vi "Main.vi"(11 "Module Admin":refnum<class "Delacor_lib_QMH_Module Admin.lvclass">) -> ()   [LabVIEW 2024, in "EtherCAT Model.lvlib"]
doc: "This template is based off of the Queued Message Handler design pattern and the Queued Message Handler project template that ships with LabVIEW.\n\nThe main difference is that the queue is private to this module and communication between modules is performed via Broadcast and Request events.\n\nRequest events are wrapped in public API methods and are handled in the Event Handling Loop (EHL) of this VI. Any module can register for Broadcast events sent by this module. The EHL generates messages based on user interface actions.\n\nThe Message Handling Loop (MHL) processes messages generated by the EHL, or by other messages. The messages are string values, so new messages can be added easily to the Message Cases case structure in the MHL. Each message cluster can also provide an optional value for Message Data, which is a variant that can be converted to whatever message-specific data is required.\n_____\nBased on DQMH Project Template 7.0.1.1316."
uses:
  EtherCAT Model.lvlib
  <vilib>/Delacor/Delacor QMH/Libraries/Module Admin_class/Delacor_lib_QMH_Module Admin.lvclass
  EtherCAT Configuration.ctl
  Module Data--cluster.ctl
  Write Context Typedef.ctl
  EtherCAT Output Data Frame.ctl
  <vilib>/Delacor/Delacor QMH/Libraries/Message Queue_class/Delacor_lib_QMH_Message Queue.lvclass/Delacor_lib_QMH_Message Queue.ctl
  Stop Argument--cluster.ctl
  <vilib>/Delacor/Delacor QMH/Libraries/Module Admin_class/Delacor_lib_QMH_Module Admin.lvclass/Delacor_lib_QMH_Module Admin.ctl
  Load Configuration Argument--cluster.ctl
  Load Configuration (Reply Payload)--cluster.ctl
  Start Connection Argument--cluster.ctl
  Start Connection (Reply Payload)--cluster.ctl
  Close Connection Argument--cluster.ctl
  Close Connection (Reply Payload)--cluster.ctl
  Write U16 Argument--cluster.ctl
  Write U16 (Reply Payload)--cluster.ctl
  Write I16 Argument--cluster.ctl
  Write I16 (Reply Payload)--cluster.ctl
  <vilib>/Utility/miscctls.llb/LVPointTypeDef.ctl
  <instrlib>/_Ackermann Automation/EtherCAT Lib/EcatLib/TypeDefs/EnumBusState.ctl
  <instrlib>/_Ackermann Automation/EtherCAT Lib/EcatLib/TypeDefs/ClusterNetworkAdapters.ctl
  <instrlib>/_Ackermann Automation/EtherCAT Lib/EcatLib/TypeDefs/ClusterTargetConnectionWin.ctl
  <vilib>/Delacor/Delacor QMH/Libraries/Message Queue_class/Delacor_lib_QMH_Enqueue Message (Single).vi
  <vilib>/Delacor/Delacor QMH/Libraries/Module Admin_class/Delacor_lib_QMH_Get External Launch.vi
  <instrlib>/_Ackermann Automation/EtherCAT Lib/EcatLib/Conversion/ConvertU16ToFrameSingle.vi
  <instrlib>/_Ackermann Automation/EtherCAT Lib/EcatLib/Conversion/ConvertI16ToFrameSingle.vi
  <vilib>/Delacor/Delacor QMH/Libraries/Message Queue_class/Delacor_lib_QMH_Message Queue.lvclass
  <instrlib>/_Ackermann Automation/EtherCAT Lib/EcatLib/EthercatLib.lvlib
panel:
  out "Setup":T1
  out "EtherCAT Ref":u64
  out "error out":errorcluster
  out "Status":string
  in  "Simulate MHL Error":bool
  in  "Simulate EHL Error":bool
  # "Other processes communicate with this Module via its Public API (wrappers for its Request Events).\n\nThis Module communicates with other processes via its Broadcast Events.\nAny process that wants to receive these messages can register for this module's Broadcast events."
  # "Local Variable"
  # "This template is for the DQMH framework. See the block diagram for more information on how to use this template."
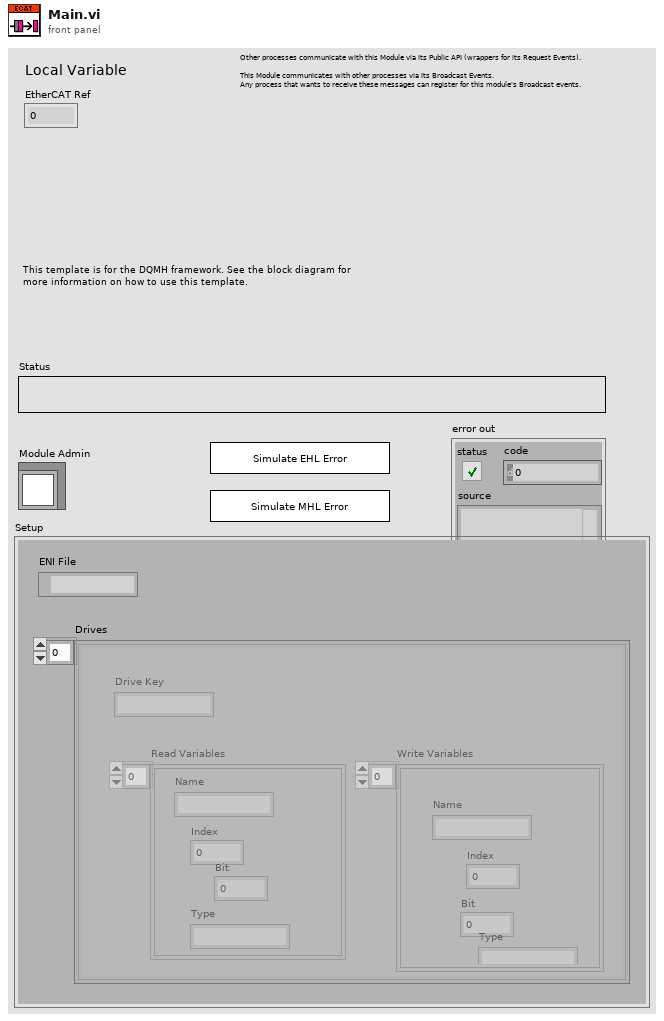
[diagram p1: front panel]
types:
  T1 = typedef "EtherCAT Configuration.ctl" = cluster{"ENI File":path, "Drives":cluster{"Drive Key":string, "Read Variables":cluster{"Name":string, "Index":i32, "Bit":u8, "Type":string}[], "Write Variables":cluster{"Name":string, "Index":i32, "Bit":u8, "Type":string}[]}[]}
  T2 = typedef "EtherCAT Model.lvlib/Request Events--cluster.ctl" = cluster{"Stop Module":refnum<user-event>, "Show Panel":refnum<user-event>, "Hide Panel":refnum<user-event>, "Get Module Execution Status":refnum<user-event>, "Show Diagram":refnum<user-event>, "Load Configuration":refnum<user-event>, "Start Connection":refnum<user-event>, "Close Connection":refnum<user-event>, "Private":cluster{"Start Read Timer Loop":refnum<user-event>, "Stop Read Timer Loop":refnum<user-event>, "Read Single Frame":refnum<user-event>}, "Write U16":refnum<user-event>, "Write I16":refnum<user-event>}
  T3 = typedef "EtherCAT Model.lvlib/Module Data--cluster.ctl" = cluster{"Status":string, "Setup":T1, "EtherCAT Connection":bool, "Write Map":T4, "EtherCAT Output Frame":T5}
  T4 = typedef "EtherCAT Model.lvlib/Write Context Typedef.ctl" = map{string, cluster{"Index":i32, "Bit":u8, "Type":string}}
  T5 = typedef "EtherCAT Model.lvlib/EtherCAT Output Data Frame.ctl" = u8[]
  T6 = enum32{"invalid lock state", "Not Locked", "Locked (No Password)", "Password-protected"}
  T7 = typedef "EtherCAT Model.lvlib/Stop Argument--cluster.ctl" = cluster{"Origin":string, "Exit via Stop Module Req?":bool, "Wait for Module to stop?":bool}
  T8 = typedef "EtherCAT Model.lvlib/Load Configuration Argument--cluster.ctl" = cluster{"Setup":T1, "Wait Notifier":refnum<notifier>, "wait for reply":bool}
  T9 = typedef "EtherCAT Model.lvlib/Start Connection Argument--cluster.ctl" = cluster{"Wait Notifier":refnum<notifier>, "wait for reply":bool}
  T10 = typedef "EtherCAT Model.lvlib/Close Connection Argument--cluster.ctl" = cluster{"Wait Notifier":refnum<notifier>, "wait for reply":bool}
  T11 = typedef "EtherCAT Model.lvlib/Write U16 Argument--cluster.ctl" = cluster{"Drive":string, "Variable":string, "Data":u16, "Wait Notifier":refnum<notifier>, "wait for reply":bool}
  T12 = typedef "EtherCAT Model.lvlib/Write I16 Argument--cluster.ctl" = cluster{"Drive":string, "Variable":string, "Data":i16, "Wait Notifier":refnum<notifier>, "wait for reply":bool}
  T13 = typedef "LVPointTypeDef.ctl" = cluster{"Horizontal":i16, "Vertical":i16}
  T14 = enum32{"Invalid", "Standard", "Closed", "Hidden", "Minimized", "Maximized"}
  T15 = typedef "EtherCAT Model.lvlib/Load Configuration (Reply Payload)--cluster.ctl" = cluster{"error":errorcluster}
  T16 = typedef "EtherCAT Model.lvlib/Start Connection (Reply Payload)--cluster.ctl" = cluster{"error":errorcluster}
  T17 = typedef "EthercatLib.lvlib/ClusterTargetConnectionWin.ctl" = cluster{"Target IP":string, "RPC Port":u32}
  T18 = typedef "EthercatLib.lvlib/ClusterNetworkAdapters.ctl" = cluster{"Primary":string, "Cable Redundancy":string}
  T19 = typedef "EtherCAT Model.lvlib/Close Connection (Reply Payload)--cluster.ctl" = cluster{"error":errorcluster}
  T20 = typedef "EtherCAT Model.lvlib/Write U16 (Reply Payload)--cluster.ctl" = cluster{"error":errorcluster}
  T21 = typedef "EtherCAT Model.lvlib/Write I16 (Reply Payload)--cluster.ctl" = cluster{"error":errorcluster}
  T22 = typedef "EthercatLib.lvlib/EnumBusState.ctl" = enum16{"Init", "PreOp", "Boot", "SafeOp", "Op"}
  T23 = typedef "EthercatLib.lvlib/ClusterBusSetup.ctl" = cluster{"Count Slaves Online":u32, "Count Slaves Configured":u32, "Process Data Bytes Input":u32, "Process Data  Bytes Output":u32, "Distributed Clocks":bool, "Hot Connect":bool}
  T24 = cluster{"Drive Key":string, "Read Variables":cluster{"Name":string, "Index":i32, "Bit":u8, "Type":string}[], "Write Variables":cluster{"Name":string, "Index":i32, "Bit":u8, "Type":string}[]}[]
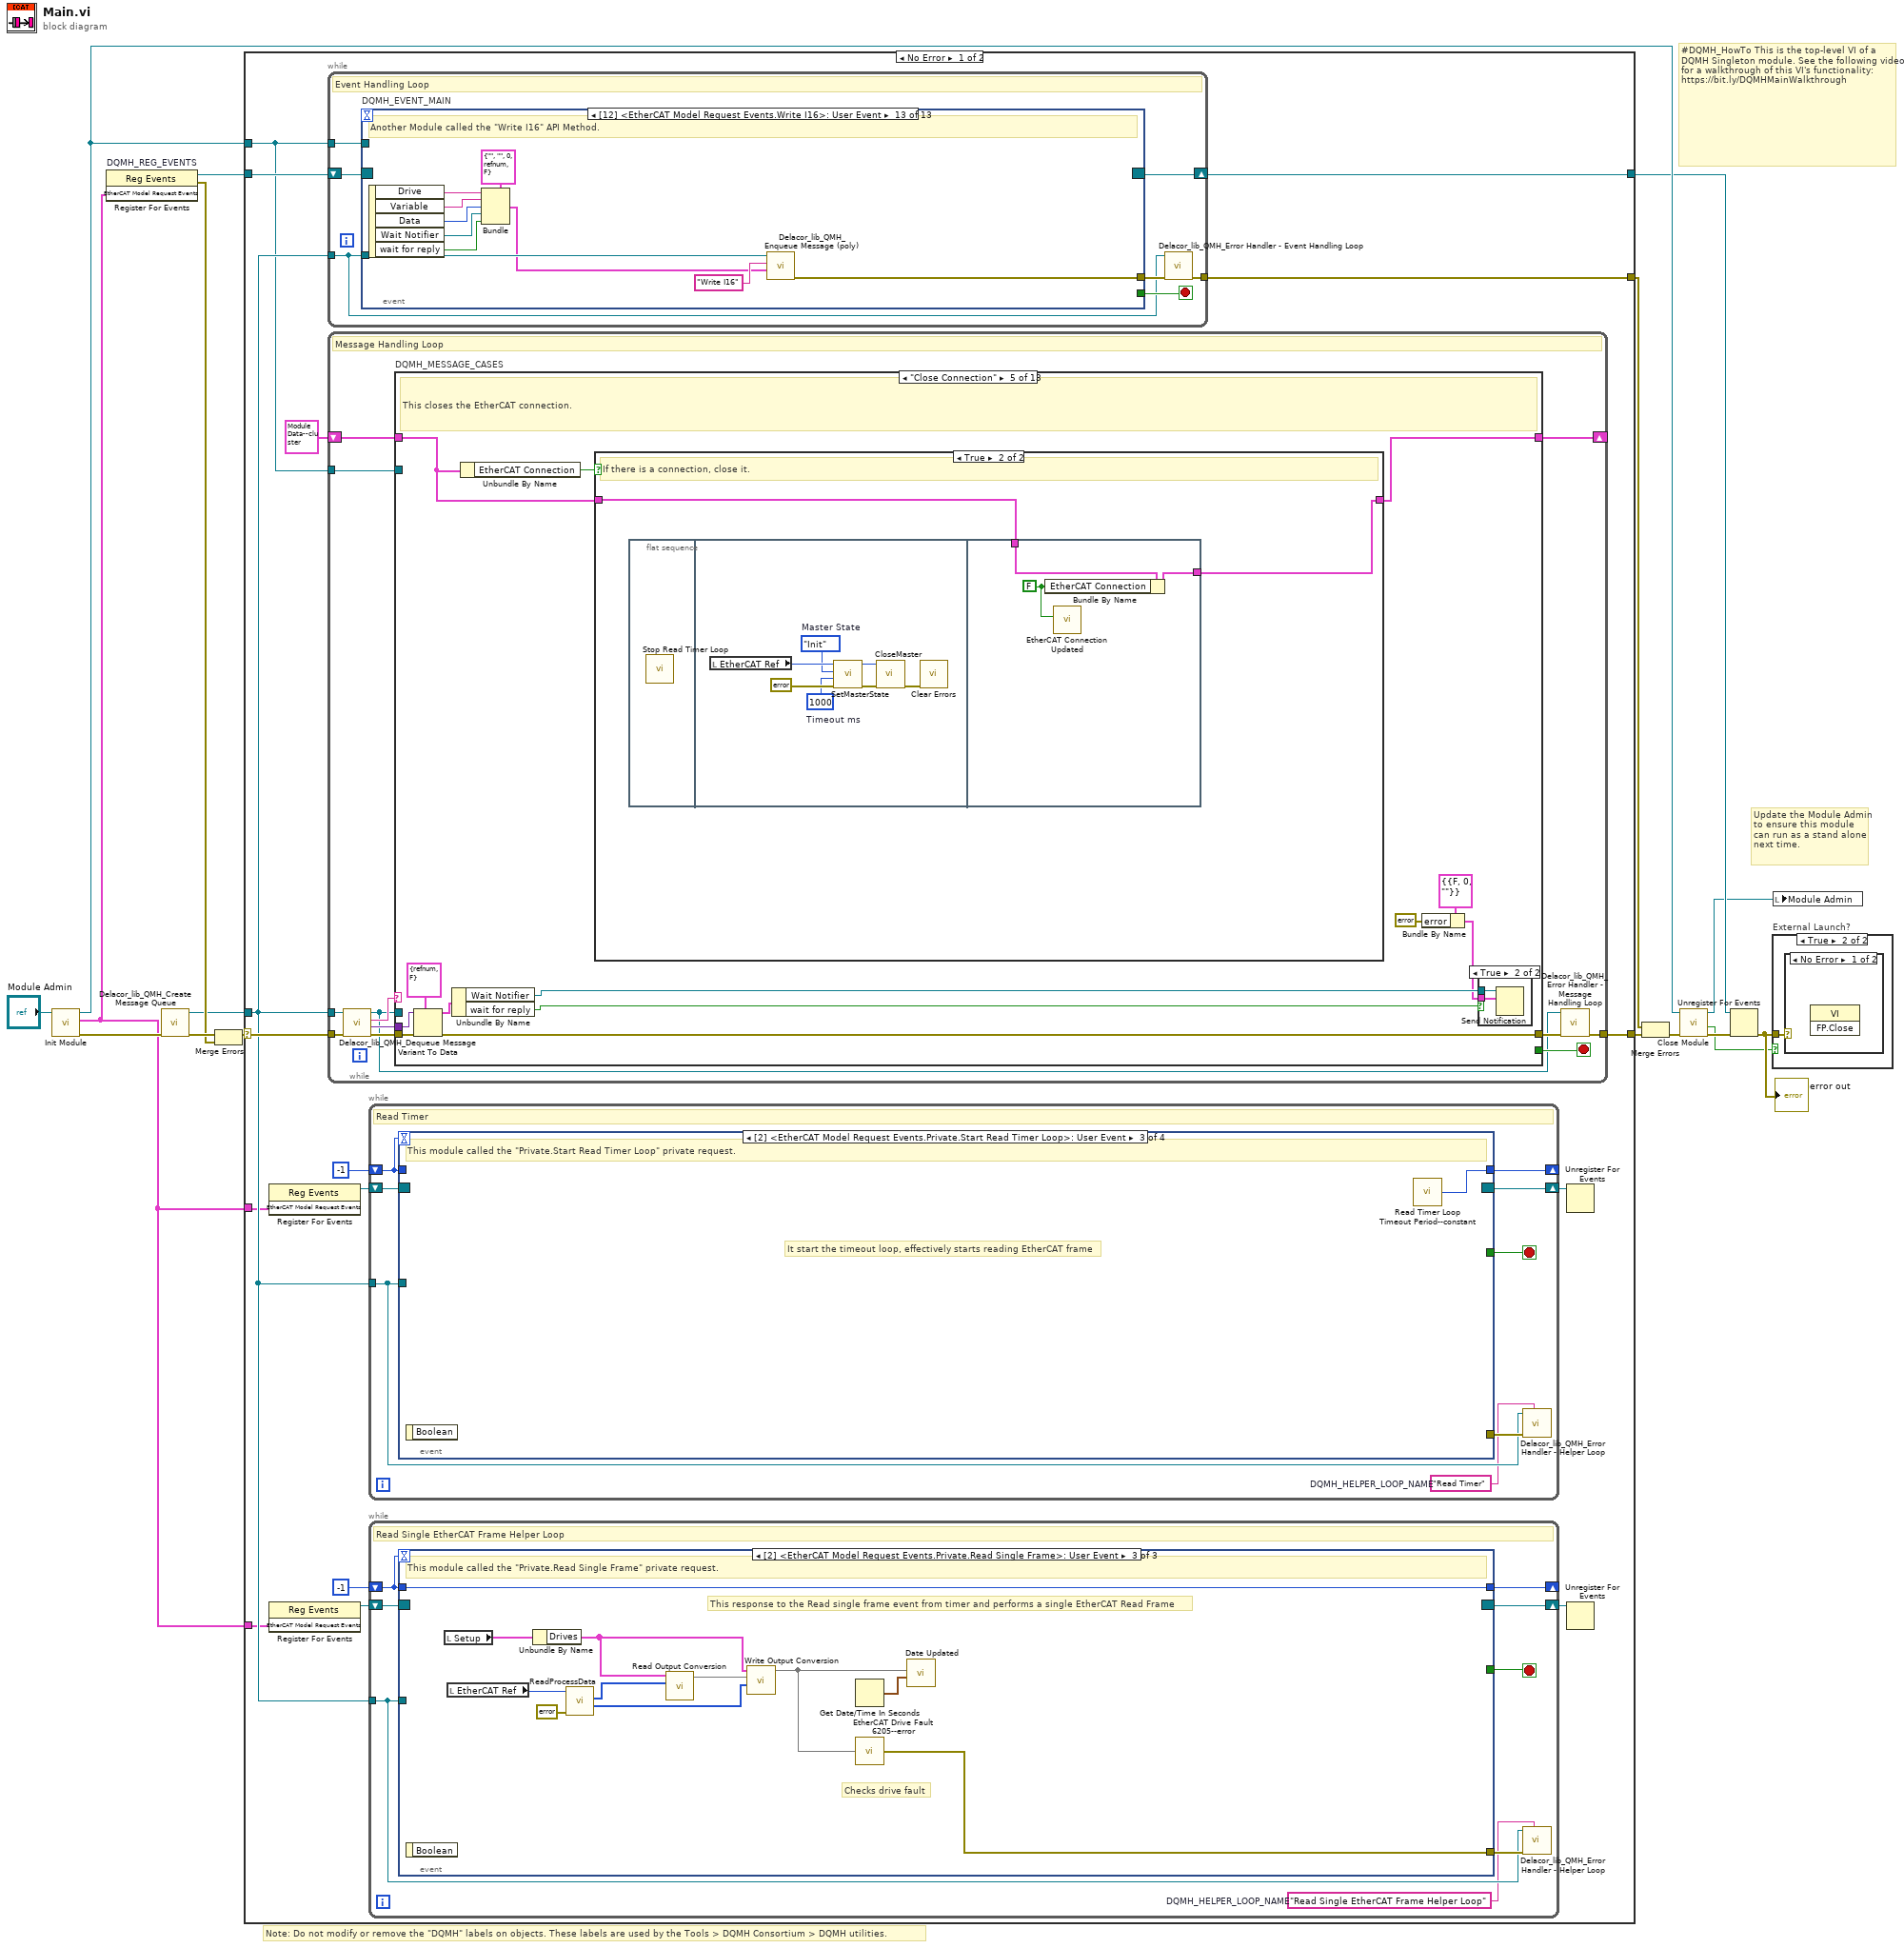
[diagram p0: block diagram]
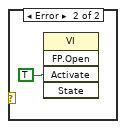
[diagram p3: hidden frame]
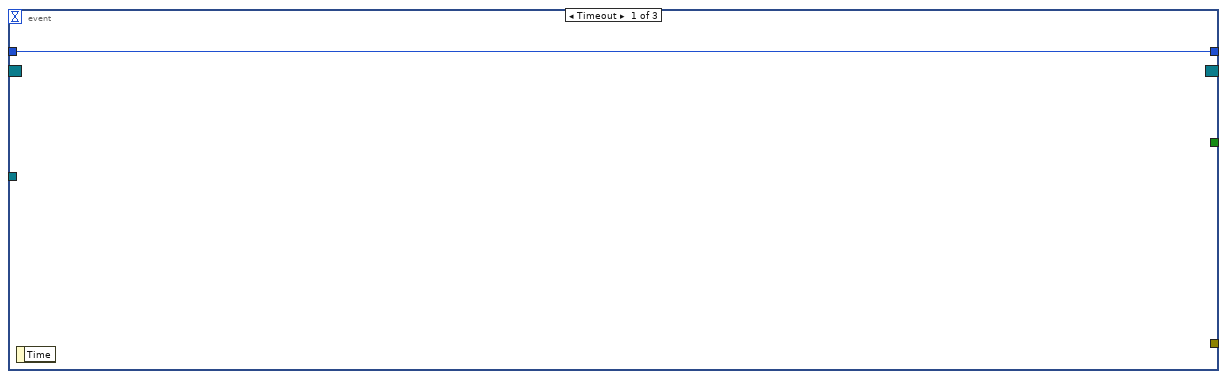
[diagram p4: hidden frame]
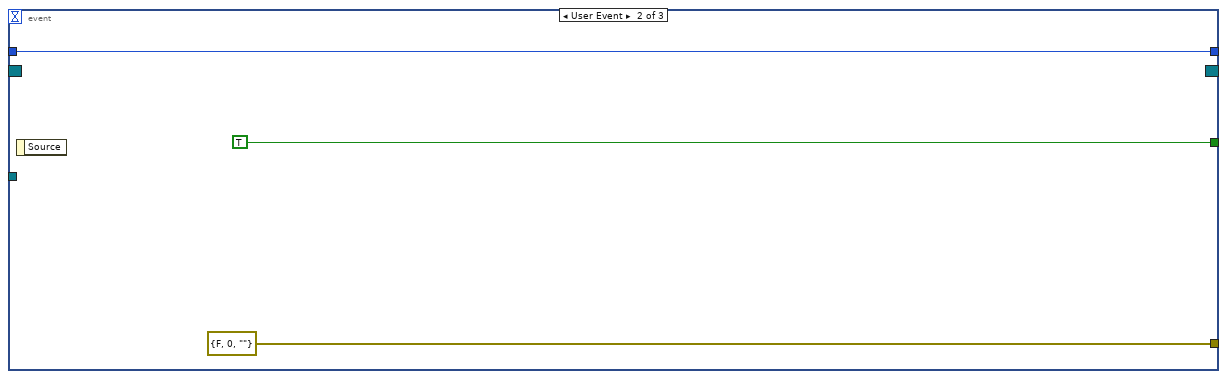
[diagram p5: hidden frame]
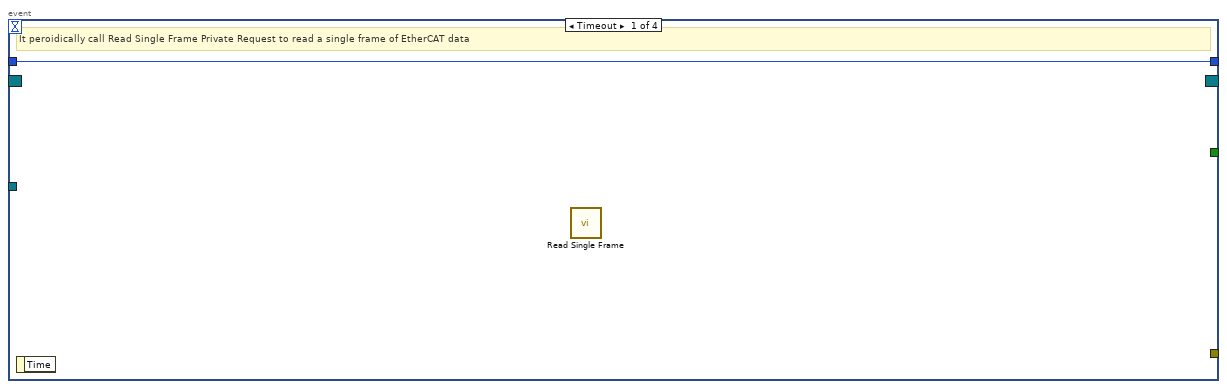
[diagram p6: hidden frame]
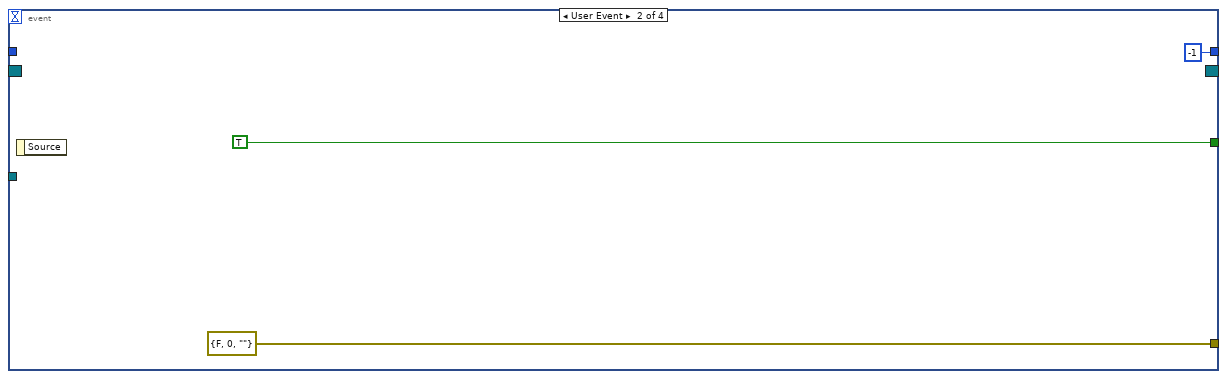
[diagram p7: hidden frame]
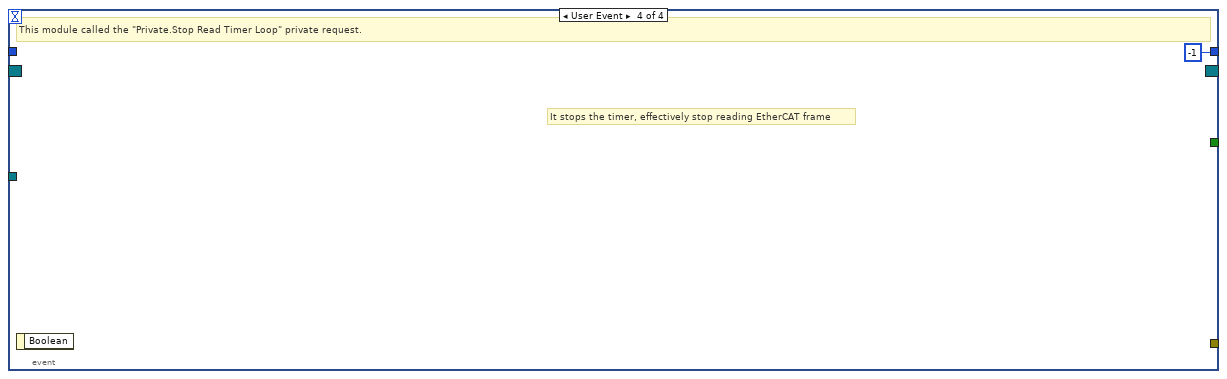
[diagram p8: hidden frame]
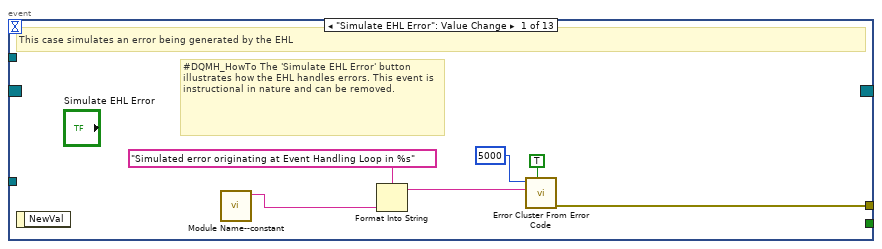
[diagram p9: hidden frame]
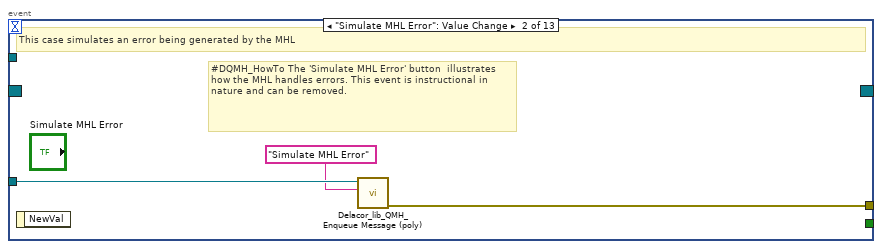
[diagram p10: hidden frame]
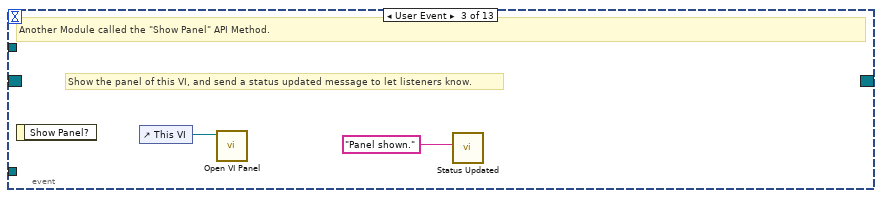
[diagram p11: hidden frame]
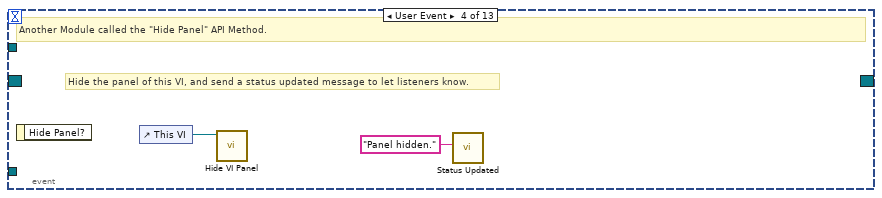
[diagram p12: hidden frame]
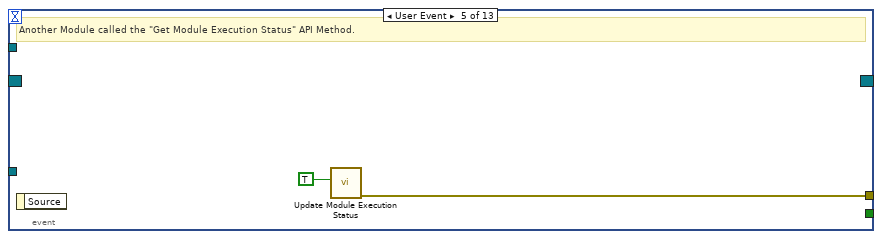
[diagram p13: hidden frame]
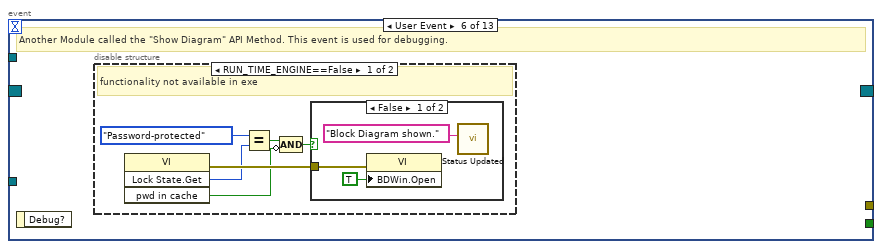
[diagram p14: hidden frame]
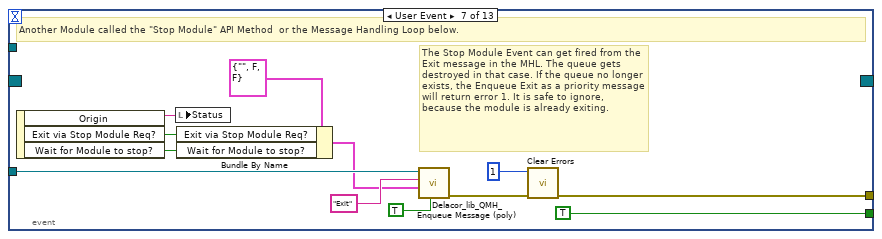
[diagram p17: hidden frame]
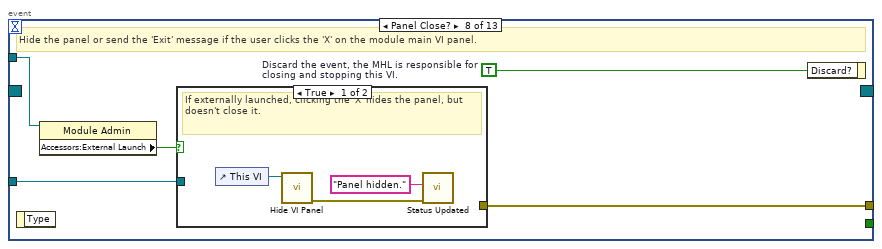
[diagram p18: hidden frame]
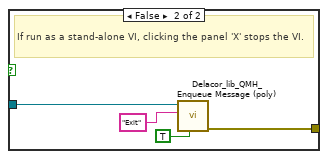
[diagram p19: hidden frame]
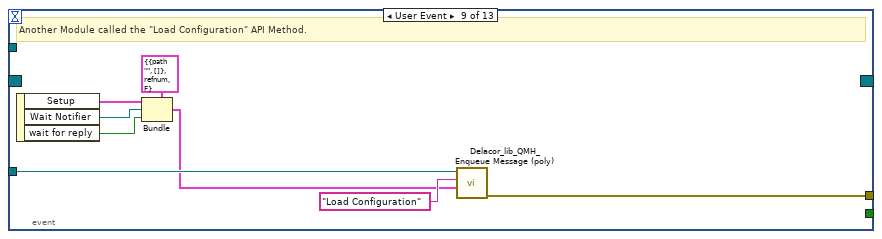
[diagram p20: hidden frame]
diagram:
  # "#DQMH_HowTo This is the top-level VI of a DQMH Singleton module. See the following video for a walkthrough of this VI's functionality: https://bit.ly/DQMHMainWalkthrough"
  # "Note: Do not modify or remove the \"DQMH\" labels on objects. These labels are used by the Tools > DQMH Consortium > DQMH utilities."
  # "Update the Module Admin to ensure this module can run as a stand alone next time."
  n1 = call "Init Module.vi"("Singleton Module Admin in"="Module Admin") -> ("error out"=w16:errorcluster, "EtherCAT Model Request Events"=w1:T2, "Singleton Module Admin out"=w8:refnum<class "Delacor_lib_QMH_Module Admin.lvclass">)  [unwired: 8 in]
  n2 = register-events "DQMH_REG_EVENTS"(w1) -> (reference out=w6:refnum<event-registration>, error out=w9:errorcluster)  [unwired: 2 in]
  n3 = call <vilib>:"Delacor_lib_QMH_Create Message Queue.vi"("error in"=w16) -> ("error out"=w11:errorcluster, "Message Queue"=w5:refnum<class "Delacor_lib_QMH_Message Queue.lvclass">)  [unwired: 9 in]
  n4 = Merge Errors(w11, w9) -> (w10:errorcluster)
  n5 = case shown="No Error" w10 {
    selector: w10 -> [w31 w489]
    tunnel: [w33 w488] -> w17
    tunnel: [w30 w487] -> w7
    tunnel: w6 -> [w28 w487]
    tunnel: w5 -> [w27 w482]
    tunnel: [w32 _] -> w14
    tunnel: w8 -> [w26 w483]
    tunnel: w1 -> [w25 _]
    tunnel: w1 -> [w21 _]
    frame No Error {
      n6 = register-events ("DQMH_HELPER_REGFOREVENTS")(w25) -> (reference out=w23:refnum<event-registration>)  [unwired: 2 in, 1 out]
      n7 = register-events ("DQMH_HELPER_REGFOREVENTS")(w21) -> (reference out=w19:refnum<event-registration>)  [unwired: 2 in, 1 out]
      n8 = while {
        tunnel: w27 -> [w71]
        shift-right: [w74] -> w30
        shift-left: w28 -> [w75]
        tunnel: [w76] -> w32
        tunnel: w26 -> [w72]
        stop <- w73 stop-if-true
        # "Event Handling Loop"
        n9 = event "DQMH_EVENT_MAIN" shown="[12] <EtherCAT Model Request Events.Write I16>: User Event" {
          selector: w75 -> [_ _ _ _ _ _ _ _ _ _ _ _ _]
          dyn-events: [_ _ _ _ _ _ _ _ _ _ _ _ _] -> w74
          timeout: _ -> [_ _ _ _ _ _ _ _ _ _ _ _ _]
          tunnel: [_ _ _ _ _ _ TRUE ("Discard?") _ _ _ _ _ _] -> w73
          tunnel: w71 -> [_ w85 _ _ _ _ w109 w116 w133 w140 w147 w157 w167]
          tunnel: [w83 w86 _ _ w92 _ w112 w118 w126 w134 w141 w148 w158] -> w77
          tunnel: w72 -> [_ _ _ _ _ _ _ w115 _ _ _ _ _]
          event "Simulate EHL Error": Value Change {
            # "#DQMH_HowTo The 'Simulate EHL Error' button  illustrates how the EHL handles errors. This event is instructional in nature and can be removed."
            # "This case simulates an error being generated by the EHL"
            n10 = event-data() -> ()  [unwired: 1 in, 1 out]
            n11 = call "Module Name--constant.vi"() -> ("Module Name"=w80:string)  [unwired: 11 in]
            n12 = Format Into String(format string="Simulated error originating at Event Handling Loop in %s", w80) -> (resulting string=w81:string)  [unwired: 2 in, 1 out]
            n13 = call <vilib>:"Error Cluster From Error Code.vi"("show call chain? (False)"=TRUE, "error message (\"\")"=w81, "error code (0)"=5000) -> ("error out"=w83:errorcluster)  [unwired: 6 in]
          }
          event "Simulate MHL Error": Value Change {
            # "#DQMH_HowTo The 'Simulate MHL Error' button  illustrates how the MHL handles errors. This event is instructional in nature and can be removed."
            # "This case simulates an error being generated by the MHL"
            n14 = event-data() -> ()  [unwired: 1 in, 1 out]
            n15 = call-poly <vilib>:"Delacor_lib_QMH_Enqueue Message (poly).vi"("Message"="Simulate MHL Error", "Message Queue in"=w85) -> ("error out"=w86:errorcluster)  [unwired: 8 in, 1 out]
          }
          event User Event {
            # "Show the panel of this VI, and send a status updated message to let listeners know."
            # "Another Module called the \"Show Panel\" API Method."
            n16 = event-data() -> ()  [unwired: 1 in, 1 out]
            n17 = control-ref of="This VI"() -> (w88:refnum<vi>)
            n18 = call "Open VI Panel.vi"("VI"=w88) -> ()  [unwired: 10 in, 1 out]
            n19 = call "Status Updated.vi"("Status"="Panel shown." ("format string")) -> ()  [unwired: 10 in, 1 out]
          }
          event User Event {
            # "Hide the panel of this VI, and send a status updated message to let listeners know."
            # "Another Module called the \"Hide Panel\" API Method."
            n20 = event-data() -> ()  [unwired: 1 in, 1 out]
            n21 = control-ref of="This VI"() -> (w90:refnum<vi>)
            n22 = call "Hide VI Panel.vi"("VI"=w90) -> ()  [unwired: 10 in, 1 out]
            n23 = call "Status Updated.vi"("Status"="Panel hidden." ("format string")) -> ()  [unwired: 10 in, 1 out]
          }
          event User Event {
            # "Another Module called the \"Get Module Execution Status\" API Method."
            n24 = event-data() -> ()  [unwired: 1 in, 1 out]
            n25 = call "Update Module Execution Status.vi"("Running?"=TRUE) -> ("error out"=w92:errorcluster)  [unwired: 10 in]
          }
          event User Event {
            # "Another Module called the \"Show Diagram\" API Method. This event is used for debugging."
            n26 = event-data() -> ()  [unwired: 1 in, 1 out]
            n27 = disable-structure shown="RUN_TIME_ENGINE==False" {
              frame condition #0 (active) {
                # "functionality not available in exe"
                n28 = invoke on="Invoke Node" class="VI" method="Lock State.Get"() -> (error out=w98:errorcluster, "Get Lock State"=w97:T6, "pwd in cache"=w94:bool)  [unwired: 4 in, 1 out]
                n29 = Equal?(x=T6."Password-protected", y=w97) -> (x = y?=w95:bool)
                n30 = Compound Arithmetic op=AND(w95, invert w94) -> (w93:bool)
                n31 = case shown="False" w93 {
                  tunnel: w98 -> [w101 _]
                  frame False {
                    n32 = property on="Property Node" class="VI"(error in=w101, "BDWin.Open"=TRUE ("Block Diagram Window:Open")) -> ()  [unwired: 1 in, 2 out]
                    n33 = call "Status Updated.vi"("Status"="Block Diagram shown." ("format string")) -> ()  [unwired: 10 in, 1 out]
                  }
                  frame True {
                    # "Password-protected VI, and the password is not in the cache. Do not show the diagram."
                  }
                }
              }
              frame condition #1 {
              }
            }
          }
          event User Event {
            # "The Stop Module Event can get fired from the Exit message in the MHL. The queue gets destroyed in that case. If the queue no longer exists, the Enqueue Exit as a priority message will return error 1. It is safe to ignore, because the module is already exiting."
            # "Another Module called the \"Stop Module\" API Method  or the Message Handling Loop below."
            n34 = event-data() -> ("Origin"=w108:string, "Exit via Stop Module Req?"=w104:bool, "Wait for Module to stop?"=w103:bool)  [unwired: 1 in]
            n35 = local write "Status"(w108) -> ()
            n36 = Bundle By Name(cluster=T7 {"Origin"="", "Exit via Stop Module Req?"=FALSE, "Wait for Module to stop?"=FALSE} ("Stop Argument"), "Exit via Stop Module Req?"=w104, "Wait for Module to stop?"=w103) -> (w102:T7)
            n37 = call-poly <vilib>:"Delacor_lib_QMH_Enqueue Message (poly).vi"("Priority Message? (F)"=TRUE, "Message Data"=w102, "Message"="Exit", "Message Queue in"=w109) -> ("error out"=w113:errorcluster)  [unwired: 6 in, 1 out]
            n38 = call <vilib>:"Clear Errors.vi"("error in (no error)"=w113, "specific error code to clear (0: all)"=1) -> ("error out"=w112:errorcluster)  [unwired: 4 in, 1 out]
          }
          event Panel Close? {
            w117 = TRUE  # Discard the event, the MHL is responsible for closing and stopping this VI.
            # "Hide the panel or send the 'Exit' message if the user clicks the 'X' on the module main VI panel."
            n39 = event-data() -> ()  [unwired: 1 in, 1 out]
            n40 = property on="Property Node" class="Module Admin"(reference=w115) -> ("Accessors:External Launch"=w114:bool)  [unwired: 1 in, 2 out]
            n41 = case shown="True" w114 {
              tunnel: w116 -> [_ w124]
              tunnel: [_ w125] -> w118
              frame True {
                # "If externally launched, clicking the 'X' hides the panel, but doesn't close it."
                n42 = control-ref of="This VI"() -> (w121:refnum<vi>)
                n43 = call "Hide VI Panel.vi"("VI"=w121) -> ("error out"=w119:errorcluster)  [unwired: 10 in]
                n44 = call "Status Updated.vi"("error in"=w119, "Status"="Panel hidden." ("format string")) -> ()  [unwired: 9 in, 1 out]
              }
              frame False {
                # "If run as a stand-alone VI, clicking the panel 'X' stops the VI."
                n45 = call-poly <vilib>:"Delacor_lib_QMH_Enqueue Message (poly).vi"("Priority Message? (F)"=TRUE, "Message"="Exit", "Message Queue in"=w124) -> ("error out"=w125:errorcluster)  [unwired: 7 in, 1 out]
              }
            }
            n46 = event-data ("Event Filter Node")("Discard?"=w117) -> ()  [unwired: 1 in, 1 out]
          }
          event User Event {
            # "Another Module called the \"Load Configuration\" API Method."
            n47 = event-data() -> ("Setup"=w129:T1, "Wait Notifier"=w128:refnum<notifier>, "wait for reply"=w127:bool)  [unwired: 1 in]
            n48 = Bundle(cluster=T8 {"Setup"={"ENI File"=path "", "Drives"=[]}, "Wait Notifier"=refnum, "wait for reply"=FALSE} ("Load Configuration Argument"), "Setup"=w129, "Wait Notifier"=w128, "wait for reply"=w127) -> (w130:T8)
            n49 = call-poly <vilib>:"Delacor_lib_QMH_Enqueue Message (poly).vi"("Message Data"=w130, "Message"="Load Configuration", "Message Queue in"=w133) -> ("error out"=w126:errorcluster)  [unwired: 7 in, 1 out]
          }
          event User Event {
            # "Another Module called the \"Start Connection\" API Method."
            n50 = event-data() -> ("Wait Notifier"=w136:refnum<notifier>, "wait for reply"=w135:bool)  [unwired: 1 in]
            n51 = Bundle(cluster=T9 {"Wait Notifier"=refnum, "wait for reply"=FALSE} ("Start Connection Argument"), "Wait Notifier"=w136, "wait for reply"=w135) -> (w137:T9)
            n52 = call-poly <vilib>:"Delacor_lib_QMH_Enqueue Message (poly).vi"("Message Data"=w137, "Message"="Start Connection", "Message Queue in"=w140) -> ("error out"=w134:errorcluster)  [unwired: 7 in, 1 out]
          }
          event User Event {
            # "Another Module called the \"Close Connection\" API Method."
            n53 = event-data() -> ("Wait Notifier"=w143:refnum<notifier>, "wait for reply"=w142:bool)  [unwired: 1 in]
            n54 = Bundle(cluster=T10 {"Wait Notifier"=refnum, "wait for reply"=FALSE} ("Close Connection Argument"), "Wait Notifier"=w143, "wait for reply"=w142) -> (w144:T10)
            n55 = call-poly <vilib>:"Delacor_lib_QMH_Enqueue Message (poly).vi"("Message Data"=w144, "Message"="Close Connection", "Message Queue in"=w147) -> ("error out"=w141:errorcluster)  [unwired: 7 in, 1 out]
          }
          event User Event {
            # "Another Module called the \"Write U16\" API Method."
            n56 = event-data() -> ("Drive"=w153:string, "Variable"=w152:string, "Data"=w151:u16, "Wait Notifier"=w150:refnum<notifier>, "wait for reply"=w149:bool)  [unwired: 1 in]
            n57 = Bundle(cluster=T11 {"Drive"="", "Variable"="", "Data"=0, "Wait Notifier"=refnum, "wait for reply"=FALSE} ("Write U16 Argument"), "Drive"=w153, "Variable"=w152, "Data"=w151, "Wait Notifier"=w150, "wait for reply"=w149) -> (w154:T11)
            n58 = call-poly <vilib>:"Delacor_lib_QMH_Enqueue Message (poly).vi"("Message Data"=w154, "Message"="Write U16", "Message Queue in"=w157) -> ("error out"=w148:errorcluster)  [unwired: 7 in, 1 out]
          }
          event User Event {
            # "Another Module called the \"Write I16\" API Method."
            n59 = event-data() -> ("Drive"=w163:string, "Variable"=w162:string, "Data"=w161:i16, "Wait Notifier"=w160:refnum<notifier>, "wait for reply"=w159:bool)  [unwired: 1 in]
            n60 = Bundle(cluster=T12 {"Drive"="", "Variable"="", "Data"=0, "Wait Notifier"=refnum, "wait for reply"=FALSE} ("Write I16 Argument"), "Drive"=w163, "Variable"=w162, "Data"=w161, "Wait Notifier"=w160, "wait for reply"=w159) -> (w164:T12)
            n61 = call-poly <vilib>:"Delacor_lib_QMH_Enqueue Message (poly).vi"("Message Data"=w164, "Message"="Write I16", "Message Queue in"=w167) -> ("error out"=w158:errorcluster)  [unwired: 7 in, 1 out]
          }
        }
        n62 = call-dynamic "Delacor_lib_QMH_Error Handler - Event Handling Loop.vi"("error in"=w77, "Message Queue in"=w71) -> ("dup error in"=w76:errorcluster)  [unwired: 8 in, 1 out]
      }
      n63 = while {
        tunnel: w27 -> [w168]
        shift-right: [w176] -> _
        shift-left: T3 {"Status"="", "Setup"={"ENI File"=path "", "Drives"=[]}, "EtherCAT Connection"=FALSE, "Write Map"={}, "EtherCAT Output Frame"=[]} ("Data Cluster") -> [w177]
        tunnel: w31 -> [w179]
        tunnel: [w171] -> w33
        tunnel: w26 -> [w172]
        stop <- w175 stop-if-true
        # "Message Handling Loop"
        n64 = call-dynamic "Delacor_lib_QMH_Dequeue Message.vi"("error in"=w179, "Message Queue in"=w168) -> ("error out"=w178:errorcluster, "Message Data"=w173:variant, "Message"=w174:string, "Message Queue out"=w169:refnum<class "Delacor_lib_QMH_Message Queue.lvclass">)  [unwired: 6 in]
        n65 = case "DQMH_MESSAGE_CASES" shown="\"Close Connection\"" w174 {
          selector: w174 -> [_ _ _ _ _ _ _ _ _ _ _ _ w477]
          tunnel: w169 -> [_ _ _ _ _ _ _ _ _ _ w436 w465 _]
          tunnel: w178 -> [w197 w201 w215 w231 w290 w324 w380 w421 w423 w432 w443 w471 w480]
          tunnel: [w195 w201 w213 w222 w289 w315 w371 w420 w423 w431 w439 w466 w481] -> w170
          tunnel: w177 -> [w186 w200 w214 w219 w279 w307 w369 w419 w422 w429 w438 w464 w478]
          tunnel: [w185 w200 w204 w220 w278 w308 w369 w419 w422 w429 w438 w464 w478] -> w176
          tunnel: [_ _ _ _ _ _ _ _ _ _ _ w463 _] -> w175
          tunnel: w173 -> [_ _ w212 w229 w288 w322 w378 _ _ _ w437 w462 _]
          tunnel: w172 -> [w187 _ _ _ _ _ _ _ _ _ w435 w457 _]
          frame "Initialize" {
            w181 = "Initial Message" ("Initial Message")
            # "#CodeNeeded - Initialize the appearance of the front panel."
            # "#CodeNeeded - Initialize your state data here."
            # "Initialize - Any operation that needs to be done before the module can receive messages. Synchronize Caller Events.vi will inform Start Module.vi that the module has launched and is ready to receive messages. Module Did Init.vi will broadcast that the module initialized."
            n66 = call "Synchronize Caller Events.vi"("error in"=w197, "Singleton Module Admin in"=w187) -> ("error out"=w196:errorcluster, "Singleton Module Admin out"=w182:refnum<class "Delacor_lib_QMH_Module Admin.lvclass">)  [unwired: 8 in]
            n67 = property on="Property Node" class="Module Admin"(reference=w182) -> ("Accessors:External Launch"=w191:bool)  [unwired: 1 in, 2 out]
            n68 = Select(t=T14."Hidden" ("State"), s=w191, f=T14."Standard" ("State")) -> (s? t:f=w188:T14)
            n69 = call "Module Name--constant.vi"() -> ("Module Name"=w194:string)  [unwired: 11 in]
            n70 = property on="Property Node" class="VI"("Front Panel.Title"=w194) -> (reference out=w193:refnum<vi>, error out=w199:errorcluster)  [unwired: 2 in]
            n71 = call "Module Name--constant.vi"() -> ("Module Name"=w183:string)  [unwired: 11 in]
            n72 = invoke on="Invoke Node" class="VI" method="FP.Open"(reference=w193, error in=w199, "State"=w188) -> (reference out=w192:refnum<vi>, error out=w198:errorcluster)  [unwired: 2 in, 3 out]
            n73 = Bundle By Name(cluster=w186, "Status"=w181) -> (w185:T3)
            n74 = call "Module Did Init.vi"("error in"=w196, "Initialized?"=TRUE, "Origin"=w183) -> ("error out"=w195:errorcluster)  [unwired: 8 in]
            n75 = invoke on="Invoke Node" class="VI" method="FP.Center"(reference=w192, error in=w198) -> ()  [unwired: 1 in, 3 out]
            n76 = property on="Pane" class="Pane"("Origin"=T13 {"Horizontal"=0, "Vertical"=0}) -> ()  [unwired: 2 in, 2 out]
            "Status" <- w181
          }
          frame "---Module Specific---" {
            # "Separator -- The following cases handle messages specific to this Module."
          }
          frame "Load Configuration" {
            # "This loads the EtherCAT configuration."
            n77 = Variant To Data(error in=w215, type=T8 {"Setup"={"ENI File"=path "", "Drives"=[]}, "Wait Notifier"=refnum, "wait for reply"=FALSE} ("Load Configuration Argument"), Variant=w212) -> (data=w210:T8, error out=w213:errorcluster)
            n78 = Unbundle By Name(w210) -> ("Setup"=w203:T1, "Wait Notifier"=w209:refnum<notifier>, "wait for reply"=w208:bool)
            "Setup" <- w203
            n79 = call "Get Write Map.vi"("Setup"=w203) -> ("Write Map OUT"=w202:T4)
            n80 = Bundle By Name(cluster=w214, "Setup"=w203, "Write Map"=w202) -> (w204:T3)
            n81 = Bundle By Name(cluster=T15 {"error"={"status"=FALSE, "code"=0, "source"=""}} ("Load Configuration (Reply Payload)"), "error"=errorcluster {"status"=FALSE, "code"=0, "source"=""}) -> (w207:T15)
            n82 = case "DQMH_FIRE_NOTIFIER" shown="True" w208 {
              tunnel: w209 -> [_ w217]
              tunnel: w207 -> [_ w216]
              frame False {
              }
              frame True {
                n83 = Send Notification(notification=w216, notifier=w217) -> ()  [unwired: 1 in, 2 out]
              }
            }
          }
          frame "Start Connection" {
            # "This start the EtherCAT connection. It tries to open the master 5 times at max. If successful, then it bring Master to operation mode."
            n84 = Unbundle By Name(w219) -> ("EtherCAT Connection"=w218:bool)
            n85 = Variant To Data(error in=w231, type=T9 {"Wait Notifier"=refnum, "wait for reply"=FALSE} ("Start Connection Argument"), Variant=w229) -> (data=w227:T9, error out=w230:errorcluster)
            n86 = Unbundle By Name(w227) -> ("Wait Notifier"=w226:refnum<notifier>, "wait for reply"=w225:bool)
            n87 = case shown="False" w218 {
              tunnel: [w239 _] -> w221
              tunnel: w219 -> [w233 w275]
              tunnel: [w232 w275] -> w220
              frame False {
                w236 = 1000  # Timeout ms
                w238 = EnumBusState."Op"  # Master State
                # "If there is no existing connection, start connection attempts"
                n88 = call "Number of Retry Connection--constant.vi"() -> ("Number of Retry"=w242:i32)  [unwired: 1 in]
                n89 = for {
                  N: w242 -> [_]
                  tunnel: w233 -> [w267]
                  tunnel: [w264] -> w240
                  tunnel: [w261] -> w241
                  stop <- w262 stop-if-true
                  w260 = 1000  # Timeout
                  # "Stop if no error"
                  # "This tries to connect number of times until max number reached or stop when conncetion is successful"
                  n90 = Unbundle By Name(w267) -> ("Setup.ENI File"=w266:path)
                  n91 = Bundle By Name(cluster=T17 {"Target IP"="", "RPC Port"=5000} ("Master Connect Settings"), "Target IP"="localhost", "RPC Port"=u32 5000) -> (w270:T17)
                  n92 = Bundle By Name(cluster=T18 {"Primary"="", "Cable Redundancy"=""} ("Network Adapters"), "Primary"="Ethernet 2") -> (w273:T18)
                  n93 = call "Bus Cycle--constant.vi"() -> ("Bus Cycle (microsecond)"=w265:u32)  [unwired: 1 in]
                  n94 = call <instrlib>:"OpenMasterCompactWin.vi"("Timeout ms"=w260, "Network Adapters"=w273, "Bus Cycle microsec"=w265, "Path ENI File"=w266, "Target Settings"=w270) -> ("error out"=w264:errorcluster, "Task Ref out"=w261:u64)  [unwired: 3 in, 2 out]
                  n95 = Unbundle By Name(w264) -> ("status"=w263:bool)
                  n96 = Not(x=w263) -> (.not. x?=w262:bool)
                }
                n97 = call <instrlib>:"SetMasterState.vi"("Wait until set"=TRUE, "error"=w240, "Timeout ms"=w236, "Master State"=w238, "Ref Task in"=w241) -> ("error out"=w234:errorcluster, "Task Ref out"=w235:u64)  [unwired: 4 in, 1 out]
                n98 = case shown="Error .." w234 {
                  tunnel: w235 -> [w249 w255]
                  tunnel: w234 -> [w248 w256]
                  tunnel: [w247 w254] -> w239
                  tunnel: w233 -> [w251 w252]
                  tunnel: [w250 w252] -> w232
                  frame No Error {
                    w243 = TRUE ("EtherCAT Connection")
                    # "If no error, update EtherCAT Ref indicator for local variable."
                    n99 = call "Start Read Timer Loop.vi"() -> ()  [unwired: 11 in, 1 out]
                    n100 = call <instrlib>:"QueryBusSetup.vi"("error"=w248, "Task Ref in"=w249) -> ("error out"=w247:errorcluster, "Bus Setup"=w245:T23, "Task ref out"=→"EtherCAT Ref":u64)  [unwired: 5 in, 2 out]
                    n101 = call "EtherCAT Connection Updated.vi"("Connection Status"=w243) -> ()  [unwired: 10 in, 1 out]
                    n102 = call "Initialize EtherCAT Output Frame.vi"("Bus Setup"=w245) -> ("EtherCAT Output Frame"=w244:T5)
                    n103 = Bundle By Name(cluster=w251, "EtherCAT Connection"=w243, "EtherCAT Output Frame"=w244) -> (w250:T3)
                  }
                  frame Error {
                    w253 = 1000  # Timeout ms
                    w257 = EnumBusState."Init"  # Master State
                    # "If error, reset state to init and close master. Report error."
                    n104 = call <instrlib>:"SetMasterState.vi"("error"=w256, "Timeout ms"=w253, "Master State"=w257, "Ref Task in"=w255) -> ("error out"=w259:errorcluster, "Task Ref out"=w258:u64)  [unwired: 5 in, 1 out]
                    n105 = call <instrlib>:"CloseMaster.vi"("error in"=w259, "Task Ref"=w258) -> ("error out"=w254:errorcluster)  [unwired: 9 in]
                  }
                }
              }
              frame True {
                # "If existing connection exists, do nothing."
              }
            }
            n106 = Bundle By Name(cluster=T16 {"error"={"status"=FALSE, "code"=0, "source"=""}} ("Start Connection (Reply Payload)"), "error"=w221) -> (w224:T16)
            n107 = Merge Errors(w230, w221) -> (w222:errorcluster)
            n108 = case "DQMH_FIRE_NOTIFIER" shown="True" w225 {
              tunnel: w226 -> [_ w277]
              tunnel: w224 -> [_ w276]
              frame False {
              }
              frame True {
                n109 = Send Notification(notification=w276, notifier=w277) -> ()  [unwired: 1 in, 2 out]
              }
            }
          }
          frame "Close Connection" {
            # "This closes the EtherCAT connection."
            n110 = Variant To Data(error in=w290, type=T10 {"Wait Notifier"=refnum, "wait for reply"=FALSE} ("Close Connection Argument"), Variant=w288) -> (data=w286:T10, error out=w289:errorcluster)
            n111 = Unbundle By Name(w286) -> ("Wait Notifier"=w285:refnum<notifier>, "wait for reply"=w284:bool)
            n112 = Unbundle By Name(w279) -> ("EtherCAT Connection"=w280:bool)
            n113 = case shown="True" w280 {
              tunnel: w279 -> [w291 w293]
              tunnel: [w291 w292] -> w278
              frame False {
                # "If there is no connection, do nothing."
              }
              frame True {
                # "If there is a connection, close it."
                n114 = flat-sequence {
                  tunnel: w293 -> [w303]
                  tunnel: [w302] -> w292
                  frame #0 {
                    n115 = call "Stop Read Timer Loop.vi"() -> ()  [unwired: 11 in, 1 out]
                  }
                  frame #1 {
                    w295 = 1000  # Timeout ms
                    w294 = EnumBusState."Init"  # Master State
                    n116 = local read "EtherCAT Ref"() -> (w299:u64)
                    n117 = call <instrlib>:"SetMasterState.vi"("error"=errorcluster {"status"=FALSE, "code"=0, "source"=""}, "Timeout ms"=w295, "Master State"=w294, "Ref Task in"=w299) -> ("error out"=w297:errorcluster, "Task Ref out"=w298:u64)  [unwired: 5 in, 1 out]
                    n118 = call <instrlib>:"CloseMaster.vi"("error in"=w297, "Task Ref"=w298) -> ("error out"=w300:errorcluster)  [unwired: 9 in]
                    n119 = call <vilib>:"Clear Errors.vi"("error in (no error)"=w300) -> ()  [unwired: 5 in, 2 out]
                  }
                  frame #2 {
                    w301 = FALSE ("EtherCAT Connection")
                    n120 = Bundle By Name(cluster=w303, "EtherCAT Connection"=w301) -> (w302:T3)
                    n121 = call "EtherCAT Connection Updated.vi"("Connection Status"=w301) -> ()  [unwired: 10 in, 1 out]
                  }
                }
              }
            }
            n122 = Bundle By Name(cluster=T19 {"error"={"status"=FALSE, "code"=0, "source"=""}} ("Close Connection (Reply Payload)"), "error"=errorcluster {"status"=FALSE, "code"=0, "source"=""}) -> (w283:T19)
            n123 = case "DQMH_FIRE_NOTIFIER" shown="True" w284 {
              tunnel: w285 -> [_ w305]
              tunnel: w283 -> [_ w304]
              frame False {
              }
              frame True {
                n124 = Send Notification(notification=w304, notifier=w305) -> ()  [unwired: 1 in, 2 out]
              }
            }
          }
          frame "Write U16" {
            # "This writes U16 data to EtherCAT Data Frame"
            n125 = Variant To Data(error in=w324, type=T11 {"Drive"="", "Variable"="", "Data"=0, "Wait Notifier"=refnum, "wait for reply"=FALSE} ("Write U16 Argument"), Variant=w322) -> (data=w320:T11, error out=w323:errorcluster)
            n126 = Unbundle By Name(w307) -> ("EtherCAT Connection"=w314:bool)
            n127 = Unbundle By Name(w320) -> ("Drive"=w311:string, "Variable"=w312:string, "Data"=w309:u16, "Wait Notifier"=w319:refnum<notifier>, "wait for reply"=w318:bool)
            n128 = call <vilib>:"Space Constant.vi"() -> ("String"=w313:string)
            n129 = Concatenate Strings(w311, w313, w312) -> (w310:string)
            n130 = case shown="True" w314 {
              tunnel: w310 -> [_ w332]
              tunnel: w309 -> [_ w327]
              tunnel: [w326 w329] -> w308
              tunnel: w307 -> [w326 w330]
              tunnel: [w325 w328] -> w306
              frame False {
                # "If there is no connection, report error"
                n131 = call "No EtherCAT Connection 6202--error.vi"() -> ("error out"=w325:errorcluster)  [unwired: 1 in]
              }
              frame True {
                # "If there is a data connection. Proceed."
                n132 = Unbundle By Name(w330) -> ("Write Map"=w334:T4)
                n133 = Look In Map(map=w334, key=w332) -> (key not found?=w333:bool, value=w331:cluster{"Index":i32, "Bit":u8, "Type":string})  [unwired: 1 in]
                n134 = case shown="False" w333 {
                  tunnel: w331 -> [w344 _]
                  tunnel: w330 -> [w338 w360]
                  tunnel: [w337 w360] -> w329
                  tunnel: [w336 w359] -> w328
                  tunnel: w327 -> [w335 _]
                  frame False {
                    # "Variable is correct, check data type"
                    n135 = Unbundle By Name(w344) -> ("Bit"=w341:u8, "Index"=w340:i32, "Type"=w343:string)
                    n136 = Equal?(x=w343, y="UINT16") -> (x = y?=w339:bool)
                    n137 = case shown="True" w339 {
                      tunnel: w341 -> [_ w350]
                      tunnel: w340 -> [_ w349]
                      tunnel: w338 -> [w346 w356]
                      tunnel: [w346 w355] -> w337
                      tunnel: [w345 w348] -> w336
                      tunnel: w335 -> [_ w353]
                      frame False {
                        # "Wrong data type, do nothing, report error"
                        n138 = call "Incorrect EtherCAT Data type 6204--error.vi"() -> ("error out"=w345:errorcluster)  [unwired: 1 in]
                      }
                      frame True {
                        # "If data type is correct, convert data and write to single frame"
                        n139 = Unbundle By Name(w356) -> ("EtherCAT Output Frame"=w354:T5)
                        n140 = call-poly <instrlib>:"ConvertToFrameSingle.vi"("Bit Index"=w350, "U16"=w353, "Byte Index"=w349, "Acquisition Data"=w354) -> ("Acquisition Data out"=w351:u8[])  [unwired: 7 in]
                        n141 = local read "EtherCAT Ref"() -> (w352:u64)
                        n142 = call <instrlib>:"WriteProcessData.vi"("Output Data"=w351, "Task Ref in"=w352) -> ("error out"=w348:errorcluster)  [unwired: 8 in, 1 out]
                        n143 = case shown="No Error" w348 {
                          tunnel: [TRUE ("Connection Status") w358] -> w347
                          frame No Error {
                          }
                          frame Error {
                            w358 = FALSE ("Connection Status")
                            n144 = call "EtherCAT Connection Updated.vi"("Connection Status"=w358) -> ()  [unwired: 10 in, 1 out]
                          }
                        }
                        n145 = Bundle By Name(cluster=w356, "EtherCAT Output Frame"=w351, "EtherCAT Connection"=w347) -> (w355:T3)
                      }
                    }
                  }
                  frame True {
                    # "If key is not found, report error"
                    n146 = call "Incorrect EtherCAT Variable 6203--error.vi"() -> ("error out"=w359:errorcluster)  [unwired: 1 in]
                  }
                }
              }
            }
            n147 = Bundle By Name(cluster=T20 {"error"={"status"=FALSE, "code"=0, "source"=""}} ("Write U16 (Reply Payload)"), "error"=w306) -> (w317:T20)
            n148 = Merge Errors(w323, w306) -> (w315:errorcluster)
            n149 = case "DQMH_FIRE_NOTIFIER" shown="True" w318 {
              tunnel: w319 -> [_ w362]
              tunnel: w317 -> [_ w361]
              frame False {
              }
              frame True {
                n150 = Send Notification(notification=w361, notifier=w362) -> ()  [unwired: 1 in, 2 out]
              }
            }
          }
          frame "Write I16" {
            # "This writes I16 data to EtherCAT Data Frame"
            n151 = Variant To Data(error in=w380, type=T12 {"Drive"="", "Variable"="", "Data"=0, "Wait Notifier"=refnum, "wait for reply"=FALSE} ("Write I16 Argument"), Variant=w378) -> (data=w376:T12, error out=w379:errorcluster)
            n152 = Unbundle By Name(w369) -> ("EtherCAT Connection"=w370:bool)
            n153 = Unbundle By Name(w376) -> ("Drive"=w367:string, "Variable"=w366:string, "Data"=w364:i16, "Wait Notifier"=w375:refnum<notifier>, "wait for reply"=w374:bool)
            n154 = call <vilib>:"Space Constant.vi"() -> ("String"=w368:string)
            n155 = Concatenate Strings(w367, w368, w366) -> (w365:string)
            n156 = case shown="True" w370 {
              tunnel: w365 -> [_ w388]
              tunnel: w364 -> [_ w383]
              tunnel: [w382 w385] -> _
              tunnel: w369 -> [w382 w386]
              tunnel: [w381 w384] -> w363
              frame False {
                # "If there is no connection, report error"
                n157 = call "No EtherCAT Connection 6202--error.vi"() -> ("error out"=w381:errorcluster)  [unwired: 1 in]
              }
              frame True {
                # "If there is a data connection. Proceed."
                n158 = Unbundle By Name(w386) -> ("Write Map"=w390:T4)
                n159 = Look In Map(map=w390, key=w388) -> (key not found?=w389:bool, value=w387:cluster{"Index":i32, "Bit":u8, "Type":string})  [unwired: 1 in]
                n160 = case shown="False" w389 {
                  tunnel: w387 -> [w400 _]
                  tunnel: w386 -> [w394 w416]
                  tunnel: [w393 w416] -> w385
                  tunnel: [w392 w415] -> w384
                  tunnel: w383 -> [w391 _]
                  frame False {
                    # "Variable is correct, check data type"
                    n161 = Unbundle By Name(w400) -> ("Bit"=w397:u8, "Index"=w396:i32, "Type"=w399:string)
                    n162 = Equal?(x=w399, y="INT16") -> (x = y?=w395:bool)
                    n163 = case shown="True" w395 {
                      tunnel: w397 -> [_ w406]
                      tunnel: w396 -> [_ w405]
                      tunnel: w394 -> [w402 w412]
                      tunnel: [w402 w411] -> w393
                      tunnel: [w401 w404] -> w392
                      tunnel: w391 -> [_ w409]
                      frame False {
                        # "Wrong data type, do nothing, report error"
                        n164 = call "Incorrect EtherCAT Data type 6204--error.vi"() -> ("error out"=w401:errorcluster)  [unwired: 1 in]
                      }
                      frame True {
                        # "If data type is correct, convert data and write to single frame"
                        n165 = Unbundle By Name(w412) -> ("EtherCAT Output Frame"=w410:T5)
                        n166 = call-poly <instrlib>:"ConvertToFrameSingle.vi"("Bit Index"=w406, "I16"=w409, "Byte Index"=w405, "Acquisition Data"=w410) -> ("Acquisition Data out"=w407:u8[])  [unwired: 7 in]
                        n167 = local read "EtherCAT Ref"() -> (w408:u64)
                        n168 = call <instrlib>:"WriteProcessData.vi"("Output Data"=w407, "Task Ref in"=w408) -> ("error out"=w404:errorcluster)  [unwired: 8 in, 1 out]
                        n169 = case shown="No Error" w404 {
                          tunnel: [TRUE ("Connection Status") w414] -> w403
                          frame No Error {
                          }
                          frame Error {
                            w414 = FALSE ("Connection Status")
                            n170 = call "EtherCAT Connection Updated.vi"("Connection Status"=w414) -> ()  [unwired: 10 in, 1 out]
                          }
                        }
                        n171 = Bundle By Name(cluster=w412, "EtherCAT Output Frame"=w407, "EtherCAT Connection"=w403) -> (w411:T3)
                      }
                    }
                  }
                  frame True {
                    # "If key is not found, report error"
                    n172 = call "Incorrect EtherCAT Variable 6203--error.vi"() -> ("error out"=w415:errorcluster)  [unwired: 1 in]
                  }
                }
              }
            }
            n173 = Bundle By Name(cluster=T21 {"error"={"status"=FALSE, "code"=0, "source"=""}} ("Write I16 (Reply Payload)"), "error"=w363) -> (w373:T21)
            n174 = Merge Errors(w379, w363) -> (w371:errorcluster)
            n175 = case "DQMH_FIRE_NOTIFIER" shown="True" w374 {
              tunnel: w375 -> [_ w418]
              tunnel: w373 -> [_ w417]
              frame False {
              }
              frame True {
                n176 = Send Notification(notification=w417, notifier=w418) -> ()  [unwired: 1 in, 2 out]
              }
            }
          }
          frame "---Copy This Frame---" {
            # "Duplicate this frame when creating new messages.  Change this comment in the duplicated frame to describe this message."
            n177 = Merge Errors(w421) -> (w420:errorcluster)
          }
          frame "---Exit and Error Handling---" {
            # "Separator - The following cases handle errors and exit messages."
          }
          frame "Simulate MHL Error" {
            # "#DQMH_HowTo The 'Simulate MHL Error' button  illustrates how the MHL handles errors. This event is instructional in nature and can be removed."
            # "Simulate an error occurring at the MHL"
            n178 = call "Module Name--constant.vi"() -> ("Module Name"=w425:string)  [unwired: 11 in]
            n179 = Format Into String(format string="Simulated error originating at Message Handling Loop in %s", w425) -> (resulting string=w426:string)  [unwired: 2 in, 1 out]
            n180 = call <vilib>:"Error Cluster From Error Code.vi"("show call chain? (False)"=TRUE, "error message (\"\")"=w426, "error code (0)"=5001) -> ("error out"=w430:errorcluster)  [unwired: 6 in]
            n181 = Merge Errors(w432, w430) -> (w431:errorcluster)
          }
          frame "Error" {
            # "#CodeRecommended - If the module is running in standalone mode (External Launch = FALSE), this code will pop up an error dialog and call the 'Exit' message if an error occurs. Add more fine-grained error management here."
            # "Error - Check the error message data and respond accordingly. This message is sent by the \"Error Handler\" VIs at the end of each loop in this application."
            n182 = property on="Property Node" class="Module Admin"(reference=w435) -> ("Accessors:External Launch"=w434:bool)  [unwired: 1 in, 2 out]
            n183 = Variant To Data(error in=w443, type=errorcluster {"status"=FALSE, "code"=0, "source"=""} ("error constant"), Variant=w437) -> (data=w433:errorcluster, error out=w441:errorcluster)
            n184 = local write "error out"(w433) -> ()
            n185 = call "Error Reported.vi"("Error"=w433) -> ()  [unwired: 10 in, 1 out]
            n186 = case shown="False" w434 {
              tunnel: [w448 _] -> w440
              tunnel: w436 -> [w446 _]
              tunnel: w433 -> [w447 _]
              frame False {
                n187 = disable-structure shown="Default" {
                  disable-tunnel: w447 -> [w449 _]
                  frame condition #0 (active) {
                    # "If the module is running standalone, then pop up an error dialog and call the \"Exit\" message."
                    n188 = call <vilib>:"Simple Error Handler.vi"("error in (no error)"=w449) -> ()  [unwired: 4 in, 5 out]
                  }
                  frame condition #1 {
                    # "To prevent the Simple Error Handler VI from being loaded (e.g. when deploying to a Real-Time target), add the Conditional Disable Symbol \"DQMH_Disable_SEH\" to your project and set it to TRUE."
                  }
                }
                n189 = call-poly <vilib>:"Delacor_lib_QMH_Enqueue Message (poly).vi"("Priority Message? (F)"=TRUE, "Message"="Exit", "Message Queue in"=w446) -> ("error out"=w448:errorcluster)  [unwired: 7 in, 1 out]
              }
              frame True {
                # "If the module was launched externally, calling the Error Reported broadcast VI is the only action performed by the \"Error\" message. The module's caller can then process the error appropriately."
              }
            }
            n190 = Merge Errors(w441, w440) -> (w439:errorcluster)
          }
          frame "Exit" {
            w452 = 1000  # Timeout ms
            w451 = EnumBusState."Init"  # Master State
            w461 = 91  # 91: not all Exit messages will have an argument
            w463 = TRUE  # Stop the VI
            # "Close Connection"
            # "Release the message queue reference"
            # "#CodeNeeded - Add any required cleanup code here."
            # "Exit - Exit the application."
            n191 = Variant To Data(error in=w471, type=T7 {"Origin"="", "Exit via Stop Module Req?"=FALSE, "Wait for Module to stop?"=FALSE} ("Stop Argument"), Variant=w462) -> (data=w459:T7, error out=w468:errorcluster)
            n192 = call <vilib>:"Clear Errors.vi"("error in (no error)"=w468, "specific error code to clear (0: all)"=w461) -> ("error out"=w470:errorcluster)  [unwired: 4 in, 1 out]
            n193 = control-ref of="This VI"() -> (w458:refnum<vi>)
            n194 = call-dynamic "Delacor_lib_QMH_Release Message Queue.vi"("error in"=w470, "Message Queue"=w465) -> ("error out"=w469:errorcluster)  [unwired: 9 in]
            n195 = call "Handle Exit.vi"("Stop Argument"=w459, "Admin in"=w457, "VI reference"=w458) -> ("error out"=w467:errorcluster)  [unwired: 7 in, 1 out]
            n196 = Merge Errors(w469, w467) -> (w466:errorcluster)
            n197 = call "Error Reported.vi"("Error"=w466) -> ()  [unwired: 10 in, 1 out]
            n198 = local read "EtherCAT Ref"() -> (w454:u64)
            n199 = call <instrlib>:"SetMasterState.vi"("error"=errorcluster {"status"=FALSE, "code"=0, "source"=""}, "Timeout ms"=w452, "Master State"=w451, "Ref Task in"=w454) -> ("error out"=w456:errorcluster, "Task Ref out"=w455:u64)  [unwired: 5 in, 1 out]
            n200 = call <instrlib>:"CloseMaster.vi"("error in"=w456, "Task Ref"=w455) -> ("error out"=w450:errorcluster)  [unwired: 9 in]
            n201 = call <vilib>:"Clear Errors.vi"("error in (no error)"=w450) -> ()  [unwired: 5 in, 2 out]
          }
          frame Default {
            # "'Default' case only runs if there is a message that isn't defined in any of the other cases.  Output a programming error."
            n202 = call "Module Name--constant.vi"() -> ("Module Name"=w476:string)  [unwired: 11 in]
            n203 = Format Into String(format string="The invalid message string \"%s\" was received in the Message Handling Loop for module \"%s\".", w477, w476) -> (resulting string=w472:string)  [unwired: 2 in, 1 out]
            n204 = call <vilib>:"Error Cluster From Error Code.vi"("show call chain? (False)"=TRUE, "error message (\"\")"=w472, "error code (0)"=1) -> ("error out"=w479:errorcluster)  [unwired: 6 in]
            n205 = Merge Errors(w480, w479) -> (w481:errorcluster)
          }
        }
        n206 = call-dynamic "Delacor_lib_QMH_Error Handler - Message Handling Loop.vi"("error in"=w170, "Message Queue in"=w169) -> ("dup error in"=w171:errorcluster)  [unwired: 8 in, 1 out]
      }
      n207 = while "DQMH_HELPER_LOOP" {
        shift-right: [w64] -> _
        shift-left: -1 -> [w63]
        shift-right: [w61] -> w24
        shift-left: w23 -> [w62]
        tunnel: w27 -> [w58]
        stop <- w60 stop-if-true
        w57 = "Read Timer"  # DQMH_HELPER_LOOP_NAME
        # "Read Timer"
        n208 = event "DQMH_HELPER_EVENT_STRUCTURE" shown="[2] <EtherCAT Model Request Events.Private.Start Read Timer Loop>: User Event" {
          selector: w62 -> [_ _ _ _]
          dyn-events: [_ _ _ _] -> w61
          timeout: w63 -> [_ _ _ _]
          tunnel: w63 -> [w65 _ _ _]
          tunnel: [w65 -1 ("Read Timer Timeout") w69 -1 ("Read Timer Timeout")] -> w64
          tunnel: [_ TRUE _ _] -> w60
          tunnel: [_ errorcluster {"status"=FALSE, "code"=0, "source"=""} ("error constant") _ _] -> w59
          tunnel: w58 -> [_ _ _ _]
          event Timeout {
            # "It peroidically call Read Single Frame Private Request to read a single frame of EtherCAT data"
            n209 = event-data() -> ()  [unwired: 1 in, 1 out]
            n210 = call "Read Single Frame.vi"() -> ()  [unwired: 11 in, 1 out]
          }
          event User Event {
            n211 = event-data() -> ()  [unwired: 1 in, 1 out]
          }
          event User Event {
            # "It start the timeout loop, effectively starts reading EtherCAT frame"
            # "This module called the \"Private.Start Read Timer Loop\" private request."
            n212 = event-data() -> ()  [unwired: 1 in, 1 out]
            n213 = call "Read Timer Loop Timeout Period--constant.vi"() -> ("Read Timer Timeout"=w69:i32)  [unwired: 1 in]
          }
          event User Event {
            # "It stops the timer, effectively stop reading EtherCAT frame"
            # "This module called the \"Private.Stop Read Timer Loop\" private request."
            n214 = event-data() -> ()  [unwired: 1 in, 1 out]
          }
        }
        n215 = call-dynamic "Delacor_lib_QMH_Error Handler - Helper Loop.vi"("Error Debug"=w57, "error in"=w59, "Message Queue in"=w58) -> ()  [unwired: 7 in, 2 out]
      }
      n216 = while "DQMH_HELPER_LOOP" {
        shift-right: [w41] -> _
        shift-left: -1 -> [w40]
        shift-right: [w38] -> w20
        shift-left: w19 -> [w39]
        tunnel: w27 -> [w35]
        stop <- w37 stop-if-true
        w34 = "Read Single EtherCAT Frame Helper Loop"  # DQMH_HELPER_LOOP_NAME
        # "Read Single EtherCAT Frame Helper Loop"
        n217 = event "DQMH_HELPER_EVENT_STRUCTURE" shown="[2] <EtherCAT Model Request Events.Private.Read Single Frame>: User Event" {
          selector: w39 -> [_ _ _]
          dyn-events: [_ _ _] -> w38
          timeout: w40 -> [_ _ _]
          tunnel: w40 -> [w42 w45 w56]
          tunnel: [w42 w45 w56] -> w41
          tunnel: [_ TRUE _] -> w37
          tunnel: [_ errorcluster {"status"=FALSE, "code"=0, "source"=""} ("error constant") w46] -> w36
          tunnel: w35 -> [_ _ _]
          event Timeout {
            n218 = event-data() -> ()  [unwired: 1 in, 1 out]
          }
          event User Event {
            n219 = event-data() -> ()  [unwired: 1 in, 1 out]
          }
          event User Event {
            # "Checks drive fault"
            # "This response to the Read single frame event from timer and performs a single EtherCAT Read Frame"
            # "This module called the \"Private.Read Single Frame\" private request."
            n220 = event-data() -> ()  [unwired: 1 in, 1 out]
            n221 = local read "Setup"() -> (w53:T1)
            n222 = local read "EtherCAT Ref"() -> (w55:u64)
            n223 = Unbundle By Name(w53) -> ("Drives"=w49:T24)
            n224 = call <instrlib>:"ReadProcessData.vi"("error in"=errorcluster {"status"=FALSE, "code"=0, "source"=""}, "Task Ref in"=w55) -> ("Process Data Output"=w48:u8[], "Process Data Input"=w52:u8[])  [unwired: 4 in, 4 out]
            n225 = call "Read Output Conversion.vi"("Process Data Input"=w52, "Drives"=w49) -> ("Map"=w50:map{string, dbl})  [unwired: 9 in]
            n226 = call "Write Output Conversion.vi"("Process Data Output"=w48, "Map IN"=w50, "Drives"=w49) -> ("Map OUT"=w47:map{string, dbl})  [unwired: 8 in]
            n227 = Get Date/Time In Seconds() -> (seconds since 1Jan1904=w51:timestamp)
            n228 = call "EtherCAT Drive Fault 6205--error.vi"("Map"=w47) -> ("error out"=w46:errorcluster)
            n229 = call "Date Updated.vi"("Time Stamp"=w51, "System State"=w47) -> ()  [unwired: 9 in, 1 out]
          }
        }
        n230 = call-dynamic "Delacor_lib_QMH_Error Handler - Helper Loop.vi"("Error Debug"=w34, "error in"=w36, "Message Queue in"=w35) -> ()  [unwired: 7 in, 2 out]
      }
      n231 = Unregister For Events(event registration refnum=w24) -> ()  [unwired: 1 in, 1 out]
      n232 = Unregister For Events(event registration refnum=w20) -> ()  [unwired: 1 in, 1 out]
    }
    frame Error {
      # "Synchronize Caller Events.vi will inform Start Module.vi that the module has launched and will let the code calling Start Module.vi register for broadcasts and would permit the caller receive the broadcast that an error occurred at launch time."
      n233 = call-dynamic "Delacor_lib_QMH_Release Message Queue.vi"("error in"=w489, "Message Queue"=w482) -> ("error out"=w488:errorcluster)  [unwired: 9 in]
      n234 = call "Synchronize Caller Events.vi"("Singleton Module Admin in"=w483) -> ("error out"=w490:errorcluster)  [unwired: 9 in, 1 out]
      n235 = call "Module Name--constant.vi"() -> ("Module Name"=w486:string)  [unwired: 11 in]
      n236 = Format Into String(format string="An error occurred during initialization. %s is no longer running.", w486) -> (resulting string=w484:string)  [unwired: 2 in, 1 out]
      n237 = Merge Errors(w488, w490) -> (w491:errorcluster)
      n238 = call "Error Reported.vi"("Additional Information"=w484, "Error"=w491) -> ()  [unwired: 9 in, 1 out]
    }
  }
  n239 = Merge Errors(w14, w17) -> (w13:errorcluster)
  n240 = call "Close Module.vi"("error in"=w13, "Module Admin in"=w8) -> ("error out"=w15:errorcluster, "External Launch"=w2:bool, "Module Admin out"=w3:refnum<class "Delacor_lib_QMH_Module Admin.lvclass">)  [unwired: 7 in]
  n241 = Unregister For Events(event registration refnum=w7, error in=w15) -> (error out=w12:errorcluster)
  "error out" <- w12
  n242 = case "External Launch?" shown="True" w2 {
    tunnel: w12 -> [_ w492]
    frame False {
    }
    frame True {
      n243 = case shown="No Error" w492 {
        frame No Error {
          n244 = invoke on="Invoke Node" class="VI" method="FP.Close"() -> ()  [unwired: 3 in, 3 out]
        }
        frame Error {
          n245 = invoke on="Invoke Node" class="VI" method="FP.Open"("Activate"=TRUE ("Activate?")) -> ()  [unwired: 4 in, 5 out]
        }
      }
    }
  }
  n246 = local write "Module Admin"(w3) -> ()
